vi "write_attributes.vi"(8 "error in (no error)":errorcluster, 10 "attributes":T1, 11 "SVR in":refnum<class "SVR.lvclass">) -> (0 "error out":errorcluster, 3 "SVR out":refnum<class "SVR.lvclass">)   [LabVIEW 2020, in "SVR.lvclass"]
uses:
  SVR.lvclass
  Controls/svr_attributes.ctl
  SVR.lvclass/SVR.ctl
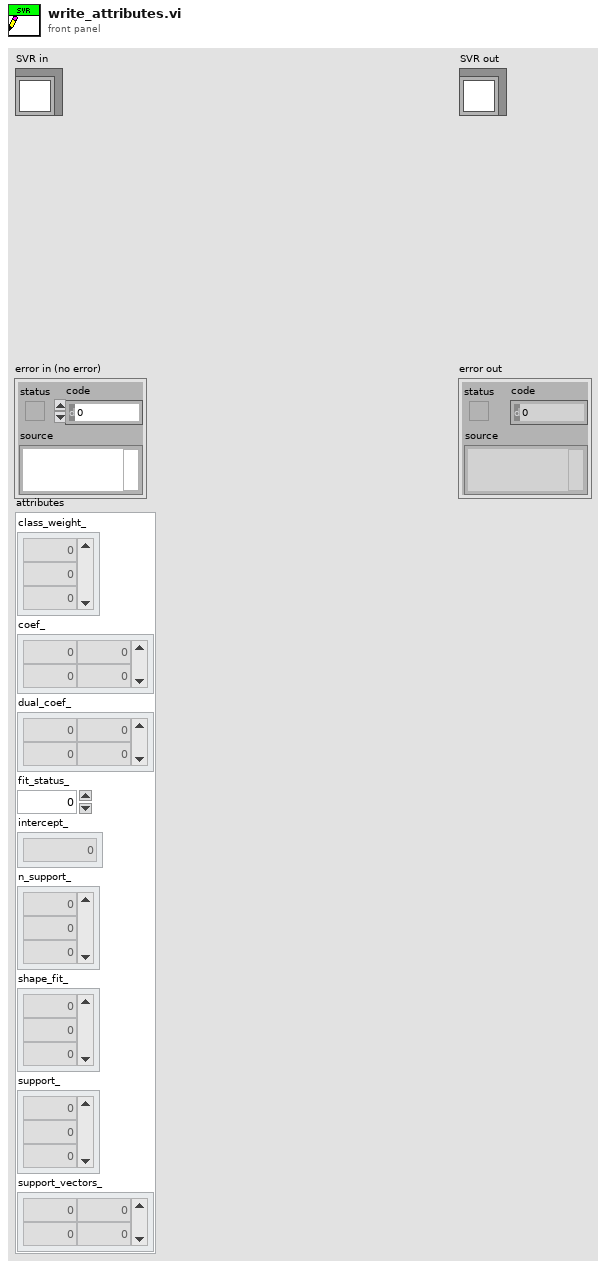
[diagram p1: front panel]
types:
  T1 = typedef "svr_attributes.ctl" = cluster{"class_weight_":dbl[], "coef_":dbl[][], "dual_coef_":dbl[][], "fit_status_":dbl, "intercept_":dbl[], "n_support_":dbl[], "shape_fit_":dbl[], "support_":dbl[], "support_vectors_":dbl[][]}
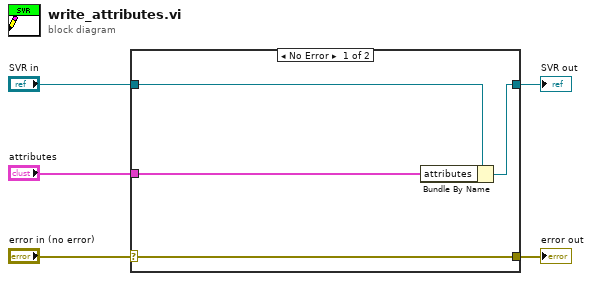
[diagram p0: block diagram]
diagram:
  n1 = case shown="No Error" "error in (no error)" {
    selector: "error in (no error)" -> [w9 w10]
    tunnel: [w9 w10] -> w4
    tunnel: [w7 w11] -> w2
    tunnel: "SVR in" -> [w8 w11]
    tunnel: "attributes" -> [w6 _]
    frame No Error {
      n2 = Bundle By Name(cluster=w8, "attributes"=w6) -> (w7:refnum<class "SVR.lvclass">)
    }
    frame Error {
    }
  }
  "error out" <- w4
  "SVR out" <- w2
